vi "ConvertPOVToJoystick.vi"(0 "POV":T1 items=["None"=-1, "POV Up"=0, "POV Up Right"=1, "POV Right"=2, "POV Down Right"=3, "POV Down"=4, "POV Down Left"=5, "POV Left"=6, "POV Up Left"=7]) -> (1 "Y-Axis":i8, 2 "X-Axis":i8)   [LabVIEW 2010, in "FTC.lvlib" / "Remote Interface.lvlib"]
uses:
  Remote Interface.lvlib
  <vilib>/FTC/FTC POVState.ctl
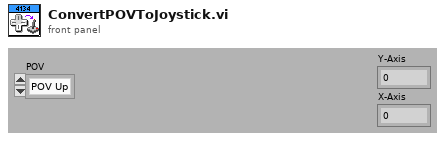
[diagram p1: front panel]
types:
  T1 = typedef "FTC POVState.ctl" = i8
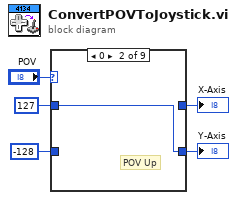
[diagram p0: block diagram]
diagram:
  n1 = case shown="0" "POV" {
    tunnel: i8 127 -> [_ w6 w7 w8 w9 _ _ _ w15]
    tunnel: i8 -128 -> [_ _ _ _ w10 w11 w12 w13 w14]
    tunnel: [_ _ w7 w8 w9 _ w12 w13 w14] -> w1
    tunnel: [_ w6 w7 _ w10 w11 w12 _ w15] -> w2
    frame -1, Default {
      # "None"
    }
    frame 0 {
      # "POV Up"
    }
    frame 1 {
      # "POV Up-Right"
    }
    frame 2 {
      # "POV Right"
    }
    frame 3 {
      # "POV Down-Right"
    }
    frame 4 {
      # "POV Down"
    }
    frame 5 {
      # "POV Down-Left"
    }
    frame 6 {
      # "POV Left"
    }
    frame 7 {
      # "POV Up-Left"
    }
  }
  "Y-Axis" <- w2
  "X-Axis" <- w1
